vi "SteinhartHartandBeta.vi"() -> ()   [LabVIEW 2014]
uses:
  <vilib>/Analysis/7linalg.llb/Solve Linear Equations (multiple right hand).vi
  <vilib>/Analysis/Matrix/Numeric/Conversions/Matrix To Array - RM.vi
  <vilib>/Utility/file.llb/Write To Spreadsheet File (DBL).vi
  <vilib>/Analysis/Matrix/NI_Matrix.lvlib
  <vilib>/Analysis/NI_AALPro.lvlib
panel:
  in  "Tab Control":T1(tab)=enum."Calculate Steinhart-Hart A, B, C"
  out "Beta TR curve":dbl[](graph)=[-0.0, 581.8712481763314, 526.0388151798995, 498.0819491960935, 479.9828996047512, 466.8251754303068, 456.5982996044473, 448.2948249748485, 441.3423551051786, 435.38642437323665, 430.193251646407, 425.60103926233916, 421.4934598824773, 417.7842527898764, 414.4077950731647, 411.31307723906616, 408.45971336220856, 405.815216830433, 403.35309074860214, 401.05145845410203, 398.8920614729931, 396.8595131880083, 394.9407340860246, 393.12451828763375, 391.4011965438649, 389.7623711637242, 388.2007052957319, 386.70975378374595, 385.28382617821114, 383.91787487394294, 382.60740306853364, 381.34838849339326, 380.1372197986173, 378.970643166712, 377.8457172535529, 376.75977495344415, 375.710390791241, 374.6953529815714, 373.71263938023725, 372.7603966983645, 371.83692246504364, 370.940649315981, 370.070131259252, 369.2240316285813, 368.40111248267976, 367.60022524838155, 366.82030243744634, 366.0603502933271, 365.3194422460667, 364.5967130716332, 363.89135366713964, 363.2026063660643, 362.5297607282293, 361.8721497482754, 361.2291464339661, 360.6001607121065, 359.9846366253532, 359.3820497878894, 358.79190507196284, 358.2137345007362, 357.64709532588654, 357.09156827095916, 356.54675592371484, 356.0122812626438, 355.487786304508, 354.97293086124216, 354.46739139583264, 353.97085996791816, 353.48304326084826, 353.0036616828054, 352.5324485353652, 352.0691492435478, 351.6135206420137, 351.16533031258945, 350.7243559687822, 350.2903848833628, 349.86321335546995, 349.44264621402704, 349.02849635455595, 348.62058430674597, 348.21873783037324, 347.8227915373804, 347.43258653812336, 347.04797010996367, 346.66879538654393, 346.2949210662247, 345.926211138291, 345.56253462565144, 345.2037653428586, 344.8497816683756, 344.5004663300996, 344.1557062032314, 343.8153921196543, 343.4794186880482, 343.1476841240253, 342.82009008962984, 342.4965415415915, 342.1769465877702, 341.86121635126904, 341.54926484173296, 341.2410088333839, 340.93636774937653, 340.63526355208745, 340.3376206389781, 340.04336574369796, 339.7524278421155, 339.4647380629868, 339.18022960299277, 338.8988376458906, 338.62049928554563, 338.34515345262304, 338.0727408447327, 337.8032038598371, 337.53648653273956, 337.27253447448675, 337.0112948145254, 336.75271614546665, 336.4967484703181, 336.2433431520536, 335.99245286539866, 335.74403155071496, 335.4980343698779, 335.2544176640438, 335.0131389132109, 334.7741566974857, 334.53743065996736, 334.30292147117166, 334.0705907949189, 333.8404012556132, 333.6123164068478, 333.3863007012713, 333.16231946165556, 332.9403388531089, 332.7203258563797, 332.5022482422011, 332.28607454662813, 332.07177404732147, 331.8593167407354, 331.6486733201691, 331.439815154642, 331.23271426855746, 331.0273433221187, 330.82367559246563, 330.6216849554996, 330.42134586836727, 330.22263335257526, 330.0255229777077, 329.82999084572305, 329.6360135758037, 329.44356828973673, 329.252632597803, 329.063184585154, 328.87520279865686, 328.68866623418717, 328.5035543243528, 328.31984692663104, 328.13752431190204, 327.95656715336406, 327.7769565158139, 327.5986738452793, 327.4217009589898, 327.24602003567173, 327.07161360615646, 326.89846454428863, 326.7265560581236, 326.55587168140374, 326.3863952653015, 326.218110970421, 326.05100325904795, 325.88505688763826, 325.7202568995373, 325.5565886179215, 325.394037638953, 325.2325898251418, 325.07223129890565, 324.9129484363227, 324.75472786106883, 324.59755643853333, 324.44142127010736, 324.28630968763844, 324.13220924804557, 323.97910772808956, 323.826993119293, 323.6758536230049, 323.5256776456054, 323.37645379384503, 323.22817087031507, 323.080817869044, 322.9343839712159, 322.788858541007, 322.64423112153656, 322.5004914309275, 322.3576293584754, 322.2156349609189, 322.0744984588126, 321.93421023299464, 321.79476082114974, 321.6561409144623, 321.51834135435826, 321.3813531293314, 321.24516737185286, 321.1097753553609, 320.9751684913277, 320.84133832640197, 320.7082765396241, 320.5759749397126, 320.4444254624184, 320.3136201679465, 320.18355123844185, 320.0542109755372, 319.9255917979634, 319.7976862392169, 319.67048694528575, 319.54398667243066, 319.41817828502013, 319.2930547534182, 319.1686091519229, 319.04483465675435, 318.9217245440905, 318.79927218815044, 318.6774710593219, 318.556314722334, 318.43579683447194, 318.3159111438341, 318.19665148762925, 318.07801179051273, 317.95998606296223, 317.84256839968947, 317.72575297808885, 317.60953405672143, 317.4939059738326, 317.378863145904, 317.2644000662373, 317.15051130356954, 317.03719150072016, 316.92443537326676, 316.8122377082511, 316.7005933629127, 316.5894972634511, 316.4789444038139, 316.3689298445119, 316.25944871146, 316.1504961948418, 316.0420675480002, 315.9341580863501, 315.82676318631553, 315.71987828428803, 315.613498875608, 315.50762051356696, 315.4022388084304, 315.2973494264815, 315.1929480890844, 315.0890305717669, 314.9855927033217, 314.8826303649267, 314.78013948928253, 314.6781160597682, 314.57655610961336, 314.4754557210876, 314.37481102470593, 314.27461819844996, 314.17487346700506, 314.07557310101214, 313.9767134163344, 313.87829077333896, 313.78030157619185, 313.6827422721674, 313.5856093509707, 313.48889934407345, 313.3926088240625, 313.29673440400103, 313.2012727368019, 313.10622051461314, 313.01157446821486, 312.917331366428, 312.82348801553405, 312.7300412587054, 312.63698797544697, 312.544325081048, 312.452049526044, 312.3601582956887, 312.26864840943585, 312.1775169204307, 312.0867609150104, 311.9963775122141, 311.9063638633016, 311.8167171512806, 311.72743459044335, 311.63851342591056, 311.5499509331843, 311.46174441770864, 311.37389121443806, 311.28638868741376, 311.19923422934727, 311.1124252612117, 311.0259592318398, 310.93983361752936, 310.8540459216557, 310.76859367429023, 310.6834744318264]
  in  "R_0":dbl=500.0
  in  "T_0":dbl=298.15
  in  "Beta":dbl=3800.0
  in  "Voltage In":dbl=5.0
  in  "Value of known resistor in voltage divider":dbl=10000.0
  in  "Save Constants to file":path
  out "Steinhart-Hart TR Curve":dbl[](graph)=[nan, 151.80696004064234, 156.17446055263414, 158.8476589741539, 160.80040810912314, 162.3483870209795, 163.6354216221259, 164.73957730157073, 165.70811965586284, 166.5719068264033, 167.3522317707158, 168.06442462448283, 168.719900274824, 169.32739394180967, 169.89374352604037, 170.42440498423161, 170.92380329083383, 171.3955782803222, 171.84276109537967, 172.26790353999704, 172.67317468934291, 173.06043424471332, 173.43128905703122, 173.78713726029042, 174.1292031445167, 174.4585650113904, 174.77617764535754, 175.0828906056407, 175.37946324054872, 175.66657710615772, 175.9448463111223, 176.21482619077779, 176.47702062497544, 176.73188824703033, 176.97984773998533, 177.2212823769831, 177.4565439319341, 177.68595606271504, 177.90981725024338, 178.128403361778, 178.34196989480762, 178.5507539482502, 178.75497595988824, 178.95484124262185, 179.1505413469328, 179.3422552726921, 179.53015054992096, 179.71438420519564, 179.8951036279541, 180.07244734892578, 180.24654574119756, 180.41752165298703, 180.58549097997476, 180.75056318401218, 180.91284176413978, 181.07242468509597, 181.229404767851, 181.38387004614586, 181.53590409253496, 181.6855863170196, 181.8329922409983, 181.97819374894985, 182.12125931999148, 182.2622542412187, 182.4012408045246, 182.53827848841465, 182.67342412617324, 182.80673206159597, 182.9382542933783, 183.06804060914095, 183.19613870997372, 183.32259432629445, 183.44745132574133, 183.57075181374904, 183.6925362273983, 183.81284342307185, 183.93171075840365, 184.04917416896188, 184.1652682400682, 184.2800262741196, 184.3934803537478, 184.50566140112218, 184.61659923367571, 184.7263226165115, 184.83485931172373, 184.9422361248502, 185.0484789486545, 185.1536128044203, 185.25766188092646, 185.3606495712573, 185.4625985075919, 185.5635305941041, 185.66346703809504, 185.76242837947225, 185.8604345186789, 185.9575047431707, 186.05365775253046, 186.14891168230375, 186.24328412663291, 186.3367921597623, 186.42945235648108, 186.52128081156695, 186.61229315828786, 186.70250458601754, 186.79192985701417, 186.88058332241025, 186.96847893745786, 187.0556302760706, 187.14205054470045, 187.22775259558694, 187.31274893941102, 187.39705175738686, 187.48067291282055, 187.56362396216414, 187.64591616559107, 187.7275604971179, 187.80856765429542, 187.88894806749104, 187.96871190878338, 188.0478691004875, 188.12642932333023, 188.20440202429188, 188.28179642413104, 188.35862152460737, 188.43488611541733, 188.51059878085616, 188.58576790621896, 188.6604016839534, 188.73450811957534, 188.80809503735796, 188.88117008580556, 188.95374074292116, 189.02581432127707, 189.09739797289788, 189.1684986939635, 189.23912332934046, 189.3092785769491, 189.37897099197346, 189.44820699092082, 189.51699285553735, 189.58533473658562, 189.65323865749048, 189.72071051785787, 189.7877560968729, 189.8543810565811, 189.9205909450584, 189.98639119947424, 190.0517871490515, 190.1167840179286, 190.18138692792598, 190.24560090122267, 190.3094308629449, 190.37288164367104, 190.43595798185552, 190.49866452617584, 190.56100583780432, 190.62298639260837, 190.68461058328197, 190.74588272141014, 190.80680703946987, 190.86738769276928, 190.92762876132733, 190.98753425169676, 191.04710809873146, 191.10635416730102, 191.16527625395415, 191.22387808853242, 191.28216333573684, 191.3401355966482, 191.39779841020317, 191.45515525462756, 191.51220954882862, 191.56896465374714, 191.625423873671, 191.68159045751187, 191.73746760004587, 191.79305844311935, 191.84836607682115, 191.90339354062277, 191.9581438244866, 192.0126198699444, 192.06682457114607, 192.1207607758802, 192.17443128656708, 192.2278388612253, 192.28098621441225, 192.33387601814033, 192.3865109027683, 192.43889345787008, 192.49102623308016, 192.5429117389177, 192.594552447589, 192.64595079376954, 192.69710917536622, 192.74802995425995, 192.79871545702972, 192.84916797565836, 192.8993897682209, 192.94938305955537, 192.99915004191746, 193.04869287561885, 193.09801368965, 193.14711458228743, 193.195997621687, 193.24466484646214, 193.29311826624837, 193.34135986225473, 193.38939158780175, 193.4372153688467, 193.48483310449643, 193.53224666750847, 193.57945790478024, 193.62646863782683, 193.67328066324788, 193.71989575318372, 193.766315655761, 193.81254209552816, 193.8585767738812, 193.90442136947956, 193.95007753865278, 193.99554691579831, 194.0408311137699, 194.0859317242581, 194.1308503181616, 194.17558844595106, 194.22014763802468, 194.26452940505592, 194.30873523833398, 194.35276661009672, 194.39662497385663, 194.44031176471938, 194.4838283996962, 194.52717627800922, 194.57035678139044, 194.6133712743744, 194.65622110458497, 194.69890760301575, 194.741432084305, 194.7837958470046, 194.82600017384385, 194.8680463319874, 194.90993557328827, 194.95166913453565, 194.99324823769746, 195.03467409015857, 195.07594788495328, 195.1170708009943, 195.1580440032964, 195.1988686431958, 195.23954585856515, 195.28007677402474, 195.32046250114888, 195.36070413866875, 195.40080277267114, 195.44075947679337, 195.48057531241423, 195.52025132884185, 195.55978856349725, 195.59918804209474, 195.63845077881908, 195.67757777649888, 195.71657002677713, 195.75542851027797, 195.79415419677125, 195.83274804533298, 195.87121100450358, 195.90954401244284, 195.94774799708222, 195.98582387627394, 196.0237725579381, 196.06159494020625, 196.09929191156317, 196.13686435098538, 196.1743131280775, 196.21163910320647, 196.2488431276325, 196.2859260436388, 196.3228886846578, 196.35973187539642, 196.3964564319579, 196.43306316196245, 196.46955286466525, 196.5059263310726, 196.54218434405593, 196.578327678464, 196.61435710123297, 196.65027337149473, 196.68607724068352, 196.72176945264002, 196.75735074371477, 196.79282184286882, 196.8281834717734, 196.8634363449074, 196.89858116965357, 196.93361864639286, 196.96854946859747, 197.00337432292207, 197.03809388929366, 197.07270884099987, 197.10721984477587]
  in  "T3":dbl=9.62
  in  "T2":dbl=20.8
  in  "T1":dbl=48.09
  in  "V3":dbl=0.4545
  in  "V2":dbl=0.283
  in  "V1":dbl=0.098
  out "A":ext=0.006587313254492917
  out "B":ext=-0.00026577273507167774
  out "C":ext=5.8849324041806116e-09
  out "R1":dbl=500204.081632653
  out "R2":dbl=166678.445229682
  out "R3":dbl=100011.00110011
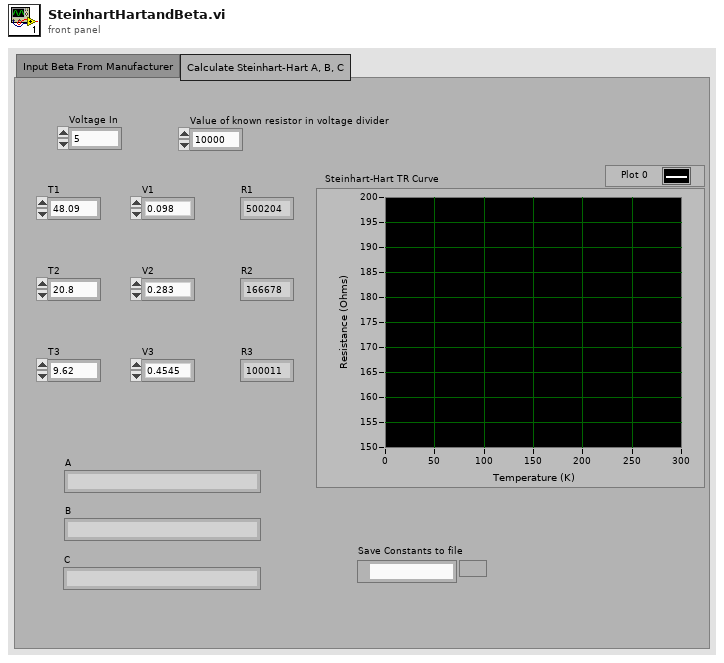
[diagram p1: front panel]
types:
  T1 = enum32{"Input Beta From Manufacturer", "Calculate Steinhart-Hart A, B, C"}
  T2 = typedef "NI_Matrix.lvlib/RealMatrix.ctl" = dbl[][]
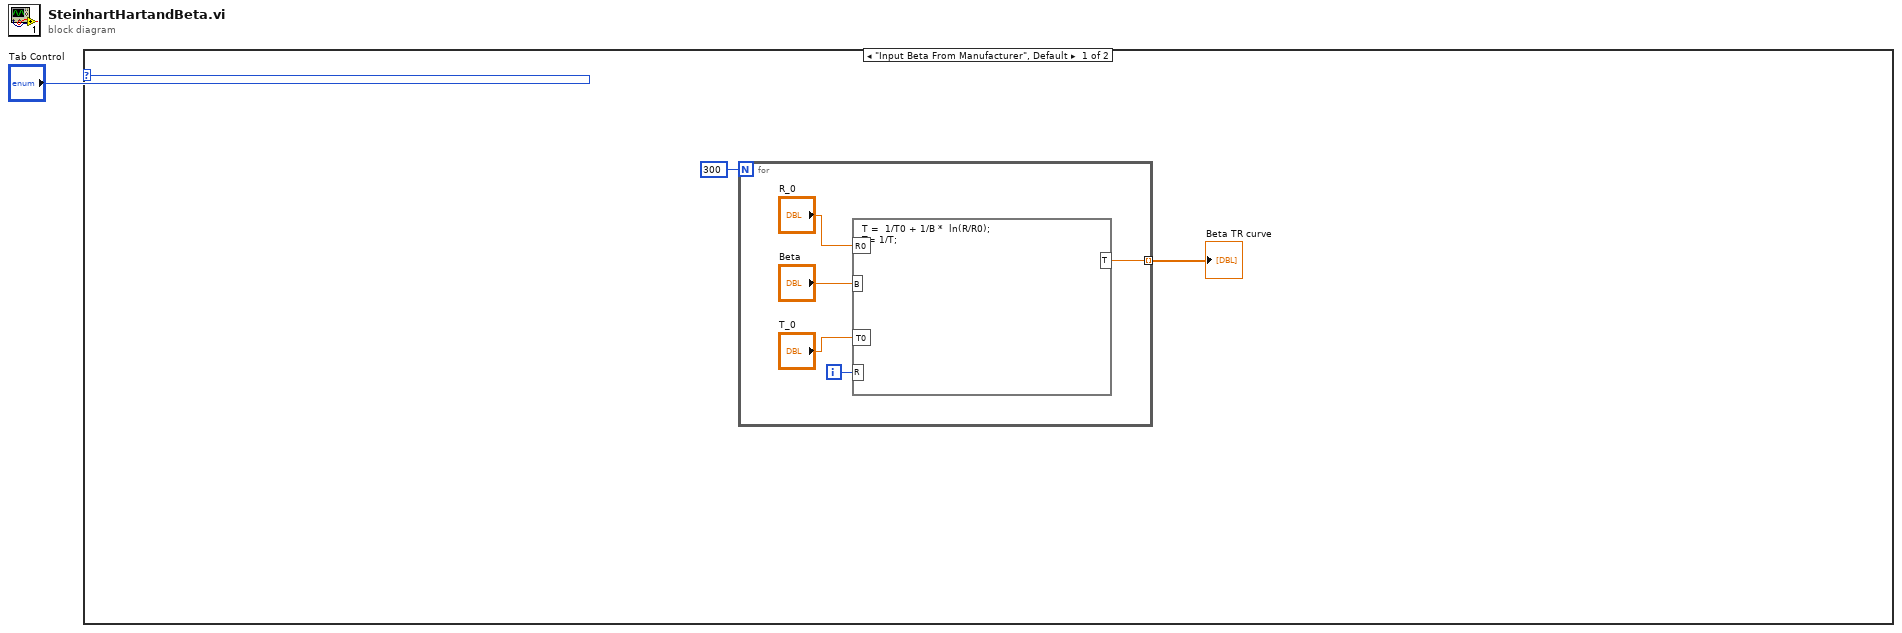
[diagram p0: block diagram]
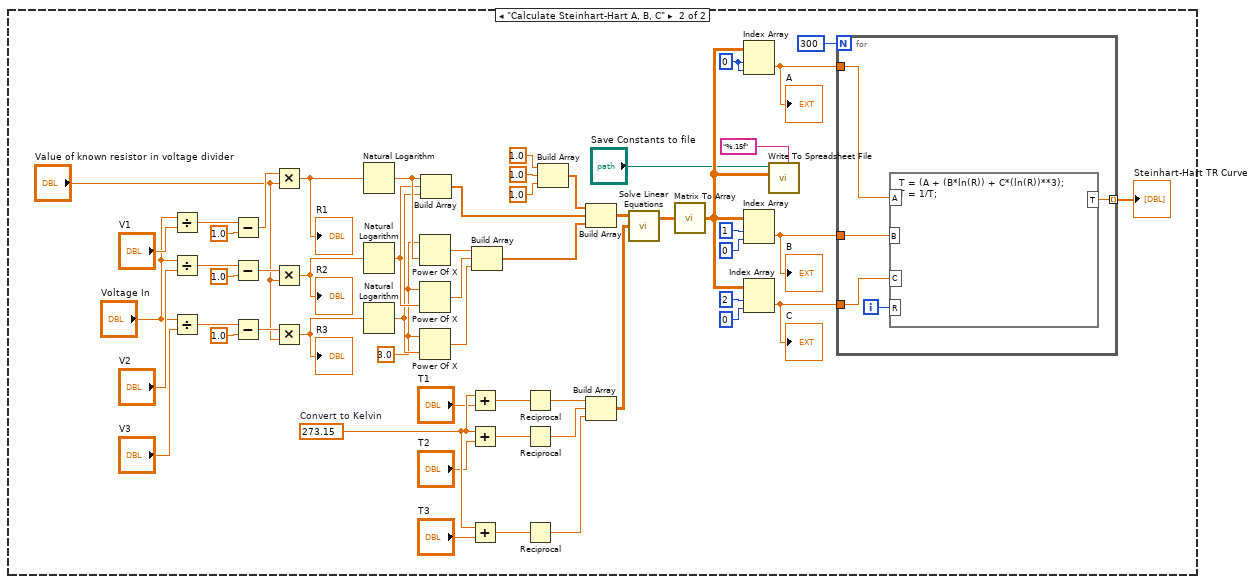
[diagram p2: hidden frame]
diagram:
  n1 = case shown="\"Input Beta From Manufacturer\", Default" "Tab Control" {
    frame "Input Beta From Manufacturer", Default {
      n2 = for {
        N: 300 -> [_]
        tunnel: [w4] -> w2 mode=indexing
        i -> [w5]
        n3 = formula code="T =  1/T0 + 1/B *  ln(R/R0);\nT= 1/T;"("R0"="R_0", "B"="Beta", "T0"="T_0", "R"=w5) -> ("T"=w4:dbl)
      }
      "Beta TR curve" <- w2
    }
    frame "Calculate Steinhart-Hart A, B, C" {
      w50 = 273.15  # Convert to Kelvin
      w51 = 0 ("index (row)")
      w58 = 3.0
      n4 = Divide(x="Voltage In", y="V1") -> (x/y=w27:dbl)
      n5 = Divide(x="Voltage In", y="V2") -> (x/y=w22:dbl)
      n6 = Divide(x="Voltage In", y="V3") -> (x/y=w17:dbl)
      n7 = Subtract(x=w27, y=1.0) -> (x-y=w26:dbl)
      n8 = Subtract(x=w22, y=1.0) -> (x-y=w21:dbl)
      n9 = Subtract(x=w17, y=1.0) -> (x-y=w16:dbl)
      n10 = Multiply(x=w26, y="Value of known resistor in voltage divider") -> (x*y=w24:dbl)
      "R1" <- w24
      n11 = Multiply(x=w21, y="Value of known resistor in voltage divider") -> (x*y=w19:dbl)
      "R2" <- w19
      n12 = Multiply(x=w16, y="Value of known resistor in voltage divider") -> (x*y=w14:dbl)
      "R3" <- w14
      n13 = Natural Logarithm(1:w24) -> (0:w61:dbl)
      n14 = Natural Logarithm(1:w19) -> (0:w60:dbl)
      n15 = Natural Logarithm(1:w14) -> (0:w59:dbl)
      n16 = Power Of X(1:w61, 2:w58) -> (0:w57:dbl)
      n17 = Power Of X(1:w60, 2:w58) -> (0:w56:dbl)
      n18 = Power Of X(1:w59, 2:w58) -> (0:w55:dbl)
      n19 = Build Array(w61, w60, w59) -> (w53:dbl[])
      n20 = Add(x=w50, y="T1") -> (x+y=w44:dbl)
      n21 = Add(x=w50, y="T2") -> (x+y=w41:dbl)
      n22 = Add(x=w50, y="T3") -> (x+y=w39:dbl)
      n23 = Build Array(w57, w56, w55) -> (w52:dbl[])
      n24 = Reciprocal(x=w44) -> (1/x=w43:dbl)
      n25 = Reciprocal(x=w41) -> (1/x=w42:dbl)
      n26 = Reciprocal(x=w39) -> (1/x=w40:dbl)
      n27 = Build Array(1.0 ("element"), 1.0 ("element"), 1.0 ("element")) -> (w54:dbl[])
      n28 = Build Array(w54, w53, w52) -> (w38:T2)
      n29 = Build Array(w43, w42, w40) -> (w45:T2)
      n30 = call-poly <vilib>:"Solve Linear Equations.vi"("Known Matrix"=w45, "Input Matrix"=w38) -> ("Solution Matrix"=w46:T2)  [unwired: 1 in, 1 out]
      n31 = call-poly <vilib>:"Matrix To Array.vi"("Real Matrix"=w46) -> ("Real 2D Array"=w13:dbl[][])
      n32 = Index Array(array=w13, index (row)=w51, index (col)=w51) -> (element=w33:dbl)
      "A" <- w33
      n33 = Index Array(array=w13, index (row)=1, index (col)=0 ("disabled index (col)")) -> (element=w32:dbl)
      "B" <- w32
      n34 = Index Array(array=w13, index (row)=2, index (col)=0 ("disabled index (col)")) -> (element=w31:dbl)
      "C" <- w31
      n35 = call-poly <vilib>:"Write To Spreadsheet File.vi"("format (%.3f)"="%.15f", "2D data"=w13, "file path (dialog if empty)"="Save Constants to file") -> ()  [unwired: 5 in, 1 out]
      n36 = for {
        N: 300 -> [_]
        tunnel: w33 -> [w69]
        tunnel: w32 -> [w68]
        tunnel: w31 -> [w67]
        tunnel: [w65] -> w29 mode=indexing
        i -> [w66]
        n37 = formula code="T = (A + (B*ln(R)) + C*(ln(R))**3);\nT = 1/T;"("A"=w69, "B"=w68, "C"=w67, "R"=w66) -> ("T"=w65:dbl)
      }
      "Steinhart-Hart TR Curve" <- w29
    }
  }
